vi "Add if New Else Append.vi"(10 "New Element":T1, 11 "Style In":T1[](array[typedef])) -> (3 "Style Out":T1[](array[typedef]))   [LabVIEW 2019, in "LSS.lvlib"]
doc: "Sort through the styles from \"New Element\" and merge them with the \"Stye In\", such that there are no duplicates and items are sorted by priority properly still.\n\n<b>Inputs:</b>\n<b>Style In</b> - Pre-parsed styles that will be merged with new input.\n<b>New Element</b> - New element that must be merged with existing LSS.\n\n<b>Outputs:</b>\n<b>Style Out</b> - Merged styles output."
uses:
  LSS.lvlib
  Controls/Style.ctl
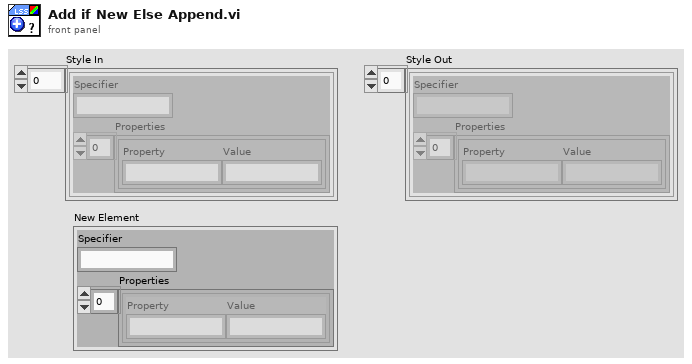
[diagram p1: front panel]
types:
  T1 = typedef "LSS.lvlib/Style.ctl" = cluster{"Specifier":string, "Properties":cluster{"Property":string, "Value":string}[]}
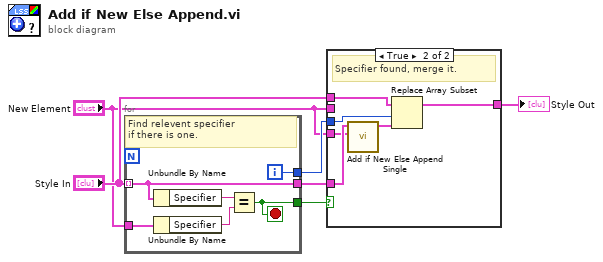
[diagram p0: block diagram]
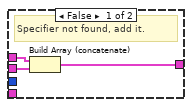
[diagram p2: hidden frame]
diagram:
  n1 = for {
    tunnel: "Style In" -> [w7] mode=indexing
    tunnel: "New Element" -> [w12]
    tunnel: [w9] -> w6
    tunnel: [w8] -> w3
    tunnel: [w7] -> w5
    i -> [w8]
    stop <- w9 stop-if-true
    # "Find relevent specifier\nif there is one."
    n2 = Unbundle By Name(w7) -> ("Specifier"=w11:string)
    n3 = Unbundle By Name(w12) -> ("Specifier"=w10:string)
    n4 = Equal?(x=w11, y=w10) -> (x = y?=w9:bool)
  }
  n5 = case shown="True" w6 {
    tunnel: w5 -> [_ w18]
    tunnel: "Style In" -> [w15 w19]
    tunnel: w3 -> [_ w21]
    tunnel: [w13 w20] -> w2
    tunnel: "New Element" -> [w14 _]
    tunnel: "New Element" -> [_ w17]
    frame False {
      # "Specifier not found, add it."
      n6 = Build Array (concatenate)(w15, w14) -> (w13:T1[])
    }
    frame True {
      # "Specifier found, merge it."
      n7 = call "Add if New Else Append Single.vi"("New Element"=w17, "Style In"=w18) -> ("Style Out"=w16:T1)  [unwired: 9 in]
      n8 = Replace Array Subset(array=w19, new element=w16, index=w21) -> (w20:T1[])
    }
  }
  "Style Out" <- w2
